vi "ep_Check Line ID.vi"(8 "error in (no error)":errorcluster, 10 "current channels":T1[](array[typedef]) {"physical channels"."channel phase" items=["Phase A (L1)", "Phase B (L2)", "Phase C (L3)", "Phase N (Neutral)"]}, 11 "voltage channels":T1[](array[typedef]) {"physical channels"."channel phase" items=["Phase A (L1)", "Phase B (L2)", "Phase C (L3)", "Phase N (Neutral)"]}) -> (0 "error out":errorcluster, 2 "number of channels":i32)   [LabVIEW 2014, in "NI_EP_Power Quality.lvlib"]
uses:
  <vilib>/addons/Electrical Power/PQ/NI_EP_Power Quality.lvlib
  <vilib>/addons/Electrical Power/PQ/Common/Controls/ep_Channels Config.ctl
  <vilib>/addons/Electrical Power/PQ/Common/Controls/ep_Channel Phase.ctl
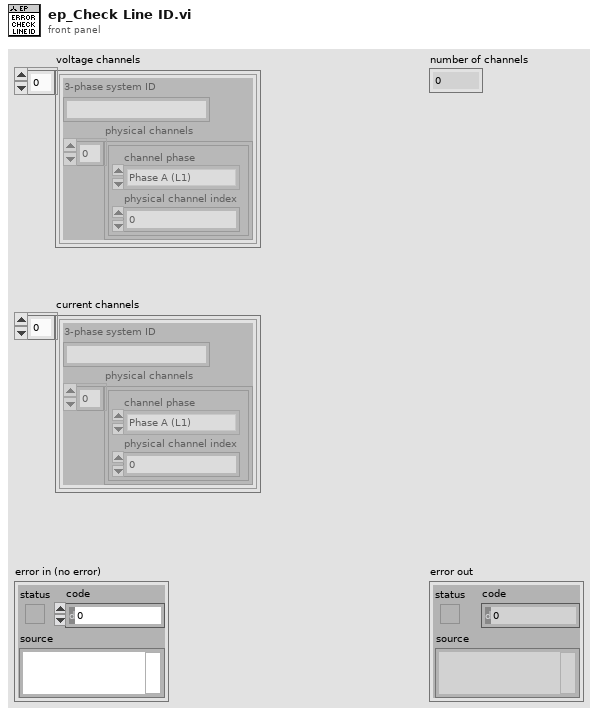
[diagram p1: front panel]
types:
  T1 = typedef "NI_EP_Power Quality.lvlib/ep_Channels Config.ctl" = cluster{"3-phase system ID":string, "physical channels":cluster{"channel phase":T2, "physical channel index":u16}[]}
  T2 = typedef "NI_EP_Power Quality.lvlib/ep_Channel Phase.ctl" = u16
  T3 = cluster{"channel phase":T2, "physical channel index":u16}[]
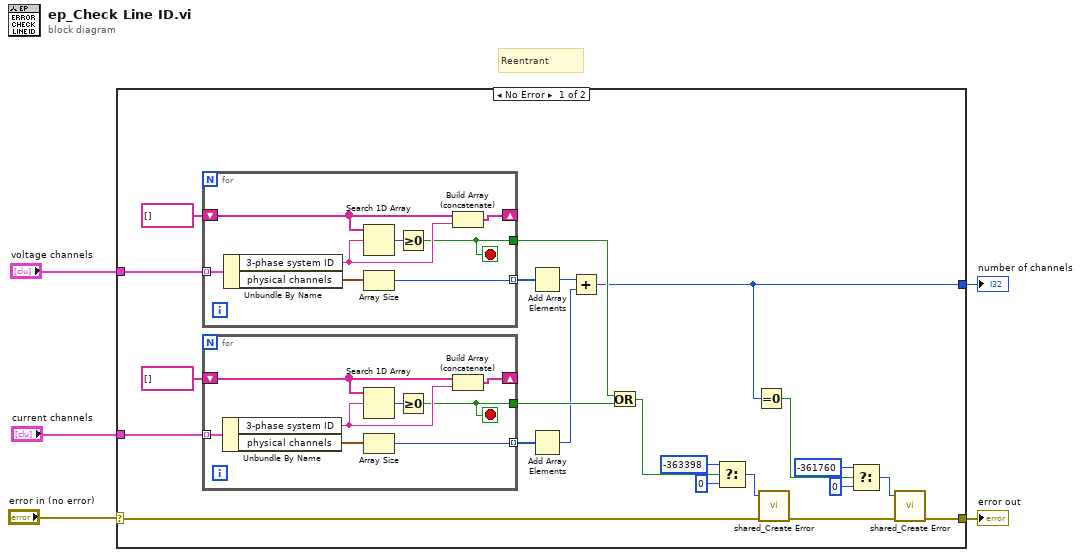
[diagram p0: block diagram]
diagram:
  # "Reentrant"
  n1 = case shown="No Error" "error in (no error)" {
    selector: "error in (no error)" -> [w19 w44]
    tunnel: "voltage channels" -> [w24 _]
    tunnel: "current channels" -> [w21 _]
    tunnel: [w11 w44] -> w4
    tunnel: [w7 _] -> w3
    frame No Error {
      n2 = for {
        tunnel: w24 -> [w41] mode=indexing
        shift-right: [w40] -> _
        shift-left: string[] [] -> [w39]
        tunnel: [w38] -> w18
        tunnel: [w36] -> w16 mode=indexing
        stop <- w38 stop-if-true
        n3 = Unbundle By Name(w41) -> ("3-phase system ID"=w42:string, "physical channels"=w37:T3)
        n4 = Search 1D Array(1D array=w39, element=w42) -> (index of element=w43:i32)  [unwired: 1 in]
        n5 = Array Size(array=w37) -> (size(s)=w36:i32)
        n6 = Greater Or Equal To 0?(x=w43) -> (x >= 0?=w38:bool)
        n7 = Build Array (concatenate)(w39, w42) -> (w40:string[])
      }
      n8 = for {
        tunnel: w21 -> [w33] mode=indexing
        shift-right: [w32] -> _
        shift-left: string[] [] -> [w31]
        tunnel: [w30] -> w17
        tunnel: [w28] -> w15 mode=indexing
        stop <- w30 stop-if-true
        n9 = Unbundle By Name(w33) -> ("3-phase system ID"=w34:string, "physical channels"=w29:T3)
        n10 = Search 1D Array(1D array=w31, element=w34) -> (index of element=w35:i32)  [unwired: 1 in]
        n11 = Array Size(array=w29) -> (size(s)=w28:i32)
        n12 = Greater Or Equal To 0?(x=w35) -> (x >= 0?=w30:bool)
        n13 = Build Array (concatenate)(w31, w34) -> (w32:string[])
      }
      n14 = Add Array Elements(numeric array=w16) -> (sum=w14:i32)
      n15 = Add Array Elements(numeric array=w15) -> (sum=w13:i32)
      n16 = Add(x=w14, y=w13) -> (x+y=w7:i32)
      n17 = Or(x=w18, y=w17) -> (x .or. y?=w20:bool)
      n18 = Select(t=-363398 ("error code (0)"), s=w20, f=0 ("error code (0)")) -> (s? t:f=w25:i32)
      n19 = Equal To 0?(x=w7) -> (x = 0?=w6:bool)
      n20 = call <vilib>:"shared_Create Error.vi"("error in (no error)"=w19, "error code (0)"=w25) -> ("error out"=w12:errorcluster)  [unwired: 9 in]
      n21 = Select(t=-361760 ("error code (0)"), s=w6, f=0 ("error code (0)")) -> (s? t:f=w8:i32)
      n22 = call <vilib>:"shared_Create Error.vi"("error in (no error)"=w12, "error code (0)"=w8) -> ("error out"=w11:errorcluster)  [unwired: 9 in]
    }
    frame Error {
    }
  }
  "error out" <- w4
  "number of channels" <- w3
